vi "Build Check Next Minor Frame.vi"(7 "Virtual Memory Unit in":refnum<class "Virtual Memory Unit.lvclass">, 8 "error in (no error)":errorcluster, 10 "Starting Address":u16 format="%04x", 11 "Major Frame in":refnum<class "Major Frame.lvclass">) -> (0 "error out":errorcluster, 2 "Next Available Address":u16 format="%04x", 3 "Major Frame out":refnum<class "Major Frame.lvclass">, 5 "Virtual Memory Unit out":refnum<class "Virtual Memory Unit.lvclass">)   [LabVIEW 2020, in "BCI-1553 API.lvlib" / "Major Frame.lvclass"]
doc: "Performs Minor Frame Completion Checks.\n\nBasically, a minor frame has completed its call chain, and now has time remaining until the next minor frame can go. This will idle and allow asynchronous messages to go out during that time.\n\nThe general premise is this:\nIs there enough time to send a high priority async?\nYes: Call the HP Async Check\nNo: Go wait for the frame timer to reach 0.\nIs there enough time to send a low priority async?\nYes: Call the LP Async Check\nNo: Go wait for the frame timer to reach 0.\nIs there enough time to send a high priority async?\nYes: Go to the HP Async call reg.\nNo: Go wait for the frame timer to reach 0.\n---\nClear GP0 and GP1 flags.\nWait for frame timer to reach 0.\nReload the minor frame time.\nStart the minor frame time.\nReturn from this subrountine."
uses:
  Major Frame.lvclass
  Dependencies/Virtual Memory Unit/Virtual Memory Unit.lvclass
  Major Frame.lvclass/Major Frame.ctl
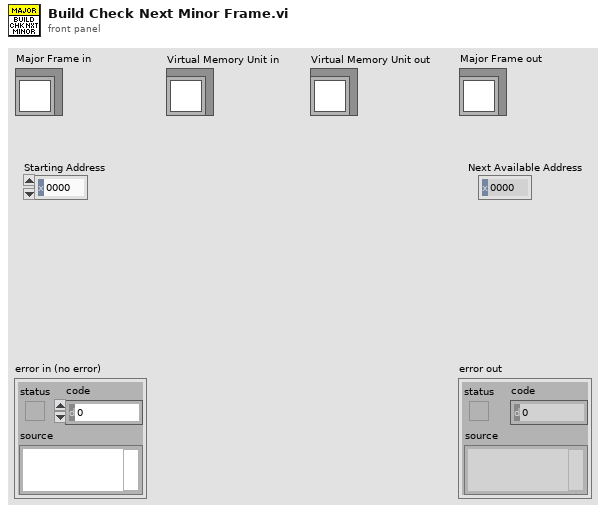
[diagram p1: front panel]
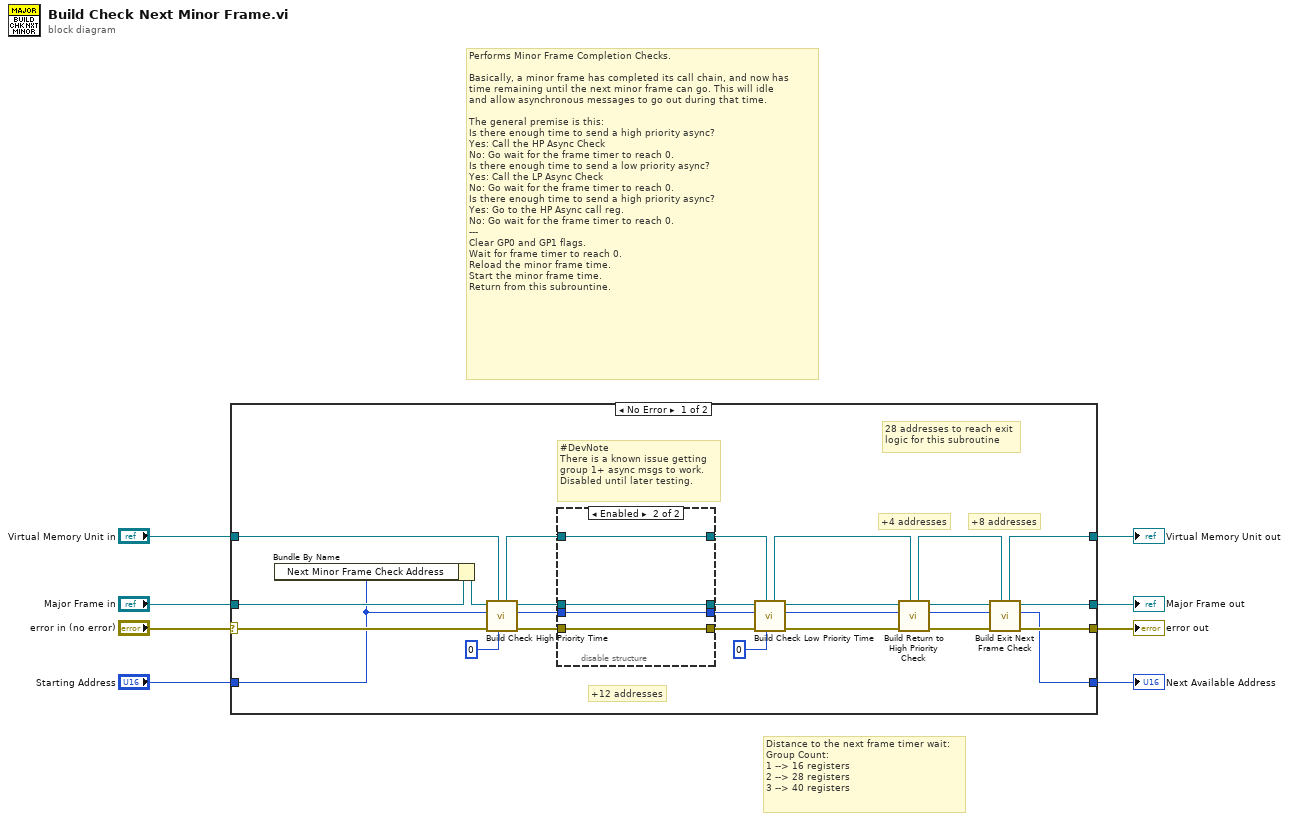
[diagram p0: block diagram]
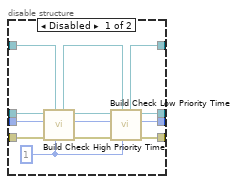
[diagram p2: hidden frame]
diagram:
  # "Distance to the next frame timer wait:\nGroup Count:\n1 --> 16 registers\n2 --> 28 registers\n3 --> 40 registers"
  # "Performs Minor Frame Completion Checks.\n\nBasically, a minor frame has completed its call chain, and now has\ntime remaining until the next minor frame can go. This will idle\nand allow asynchronous messages to go out during that time.\n\nThe general premise is this:\nIs there enough time to send a high priority async?\nYes: Call the HP Async Check\nNo: Go wait for the frame timer to reach 0.\nIs there enough time to send a low priority async?\nYes: Call the LP Async Check\nNo: Go wait for the frame timer to reach 0.\nIs there enough time to send a high priority async?\nYes: Go to the HP Async call reg.\nNo: Go wait for the frame timer to reach 0.\n---\nClear GP0 and GP1 flags.\nWait for frame timer to reach 0.\nReload the minor frame time.\nStart the minor frame time.\nReturn from this subrountine."
  n1 = case shown="No Error" "error in (no error)" {
    selector: "error in (no error)" -> [w32 w56]
    tunnel: [w28 w56] -> w7
    tunnel: [w26 w55] -> w5
    tunnel: "Major Frame in" -> [w35 w55]
    tunnel: [w25 w54] -> w4
    tunnel: "Virtual Memory Unit in" -> [w34 w54]
    tunnel: [w23 w53] -> w2
    tunnel: "Starting Address" -> [w31 w53]
    frame No Error {
      # "#DevNote\nThere is a known issue getting\ngroup 1+ async msgs to work.\nDisabled until later testing."
      # "28 addresses to reach exit\nlogic for this subroutine"
      # "+8 addresses"
      # "+4 addresses"
      # "+12 addresses"
      n2 = Bundle By Name(cluster=w35, "Next Minor Frame Check Address"=w31) -> (w33:refnum<class "Major Frame.lvclass">)
      n3 = call "Build Check High Priority Time.vi"("Group"=0, "Virtual Memory Unit in"=w34, "error in (no error)"=w32, "Starting Address"=w31, "Major Frame in"=w33) -> ("error out"=w15:errorcluster, "Next Available Address"=w16:u16, "Major Frame out"=w17:refnum<class "Major Frame.lvclass">, "Virtual Memory Unit out"=w18:refnum<class "Virtual Memory Unit.lvclass">)  [unwired: 3 in]
      n4 = disable-structure shown="Enabled" {
        disable-tunnel: w18 -> [w48 w52]
        disable-tunnel: w17 -> [w47 w51]
        disable-tunnel: w16 -> [w46 w50]
        disable-tunnel: w15 -> [w45 w49]
        disable-tunnel: [w43 w52] -> w14
        disable-tunnel: [w42 w51] -> w13
        disable-tunnel: [w39 w49] -> w12
        disable-tunnel: [w37 w50] -> w10
        frame Disabled {
          w36 = 1 ("Group")
          n5 = call "Build Check High Priority Time.vi"("Group"=w36, "Virtual Memory Unit in"=w48, "error in (no error)"=w45, "Starting Address"=w46, "Major Frame in"=w47) -> ("error out"=w40:errorcluster, "Next Available Address"=w38:u16, "Major Frame out"=w41:refnum<class "Major Frame.lvclass">, "Virtual Memory Unit out"=w44:refnum<class "Virtual Memory Unit.lvclass">)  [unwired: 3 in]
          n6 = call "Build Check Low Priority Time.vi"("Group"=w36, "Virtual Memory Unit in"=w44, "error in (no error)"=w40, "Starting Address"=w38, "Major Frame in"=w41) -> ("error out"=w39:errorcluster, "Next Available Address"=w37:u16, "Major Frame out"=w42:refnum<class "Major Frame.lvclass">, "Virtual Memory Unit out"=w43:refnum<class "Virtual Memory Unit.lvclass">)  [unwired: 3 in]
        }
        frame Enabled {
        }
      }
      n7 = call "Build Check Low Priority Time.vi"("Group"=0, "Virtual Memory Unit in"=w14, "error in (no error)"=w12, "Starting Address"=w10, "Major Frame in"=w13) -> ("error out"=w19:errorcluster, "Next Available Address"=w20:u16, "Major Frame out"=w22:refnum<class "Major Frame.lvclass">, "Virtual Memory Unit out"=w21:refnum<class "Virtual Memory Unit.lvclass">)  [unwired: 3 in]
      n8 = call "Build Return to High Priority Check.vi"("Virtual Memory Unit in"=w21, "error in (no error)"=w19, "Starting Address"=w20, "Major Frame in"=w22) -> ("error out"=w29:errorcluster, "Next Available Address"=w24:u16, "Major Frame out"=w27:refnum<class "Major Frame.lvclass">, "Virtual Memory Unit out"=w30:refnum<class "Virtual Memory Unit.lvclass">)  [unwired: 4 in]
      n9 = call "Build Exit Next Frame Check.vi"("Virtual Memory Unit in"=w30, "error in (no error)"=w29, "Starting Address"=w24, "Major Frame in"=w27) -> ("error out"=w28:errorcluster, "Next Available Address"=w23:u16, "Major Frame out"=w26:refnum<class "Major Frame.lvclass">, "Virtual Memory Unit out"=w25:refnum<class "Virtual Memory Unit.lvclass">)  [unwired: 4 in]
    }
    frame Error {
    }
  }
  "error out" <- w7
  "Major Frame out" <- w5
  "Virtual Memory Unit out" <- w4
  "Next Available Address" <- w2
